vi "traffic_light.vi"() -> ()   [LabVIEW 2019]
doc: "This is a traffic light system. It realized the output with hard device or simulated device. The light has four phases."
uses:
  <vilib>/Utility/error.llb/DialogType.ctl
  <vilib>/DAQmx/write.llb/DAQmx Write (Digital 1D Bool 1Chan 1Samp).vi
  <vilib>/DAQmx/create/channels.llb/DAQmx Create Channel (DO-Digital Output).vi
  <vilib>/DAQmx/miscellaneous.llb/DAQmx Fill In Error Info.vi
panel:
  out "Delay (ms)":u32 caption="Elapsed Time (s)"
  in  "Loop Time (ms)":u32=100 max=1000 step=50
  in  "Line(s)":tag="Dev1/port0/line0:1"
  out "Phase Time (s)":dbl caption="Elapsed Time (s)" format="%.2f"
  in  "Stop Button":bool
  out "Red":bool
  out "Yellow":bool
  out "Green":bool
  # "Note & Guide\n\nLine(s)\ndevice/port/line0:2\nmyDAQ1/port0/line0:2\n\nLoop Time (ms)\n0 - 1000\nreference: 100\n\nPhase\nGreen              3s\nYellow              2s\nRed                 5s\nRed+Yellow     1s\n\nAuthor\nYufan Dong - 06.Oct.2021"
  # "Traffic Light System"
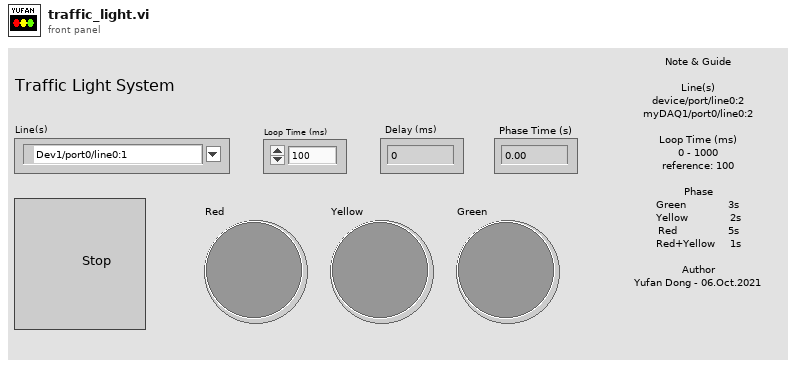
[diagram p1: front panel]
types:
  T1 = typedef "DialogType.ctl" = u16
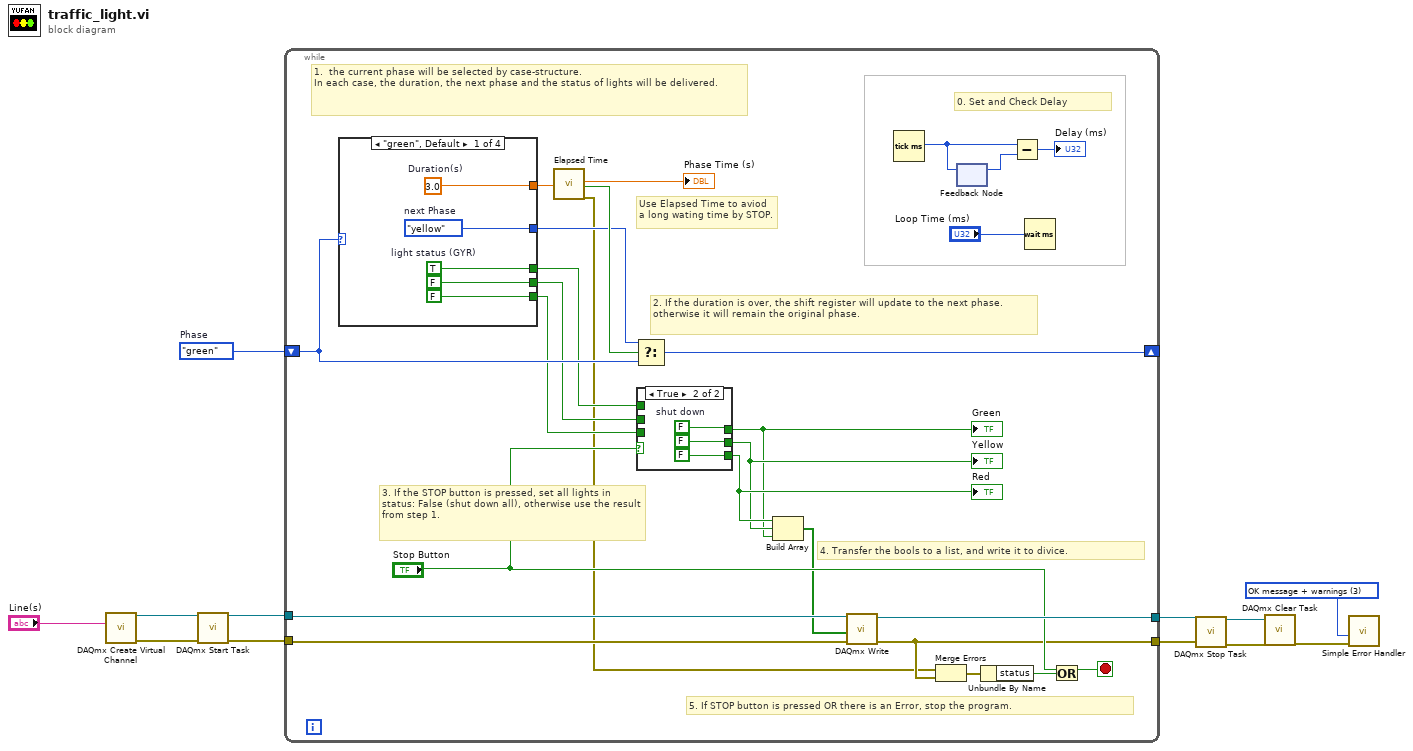
[diagram p0: block diagram]
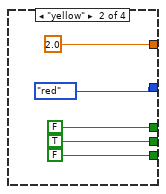
[diagram p3: hidden frame]
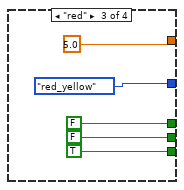
[diagram p4: hidden frame]
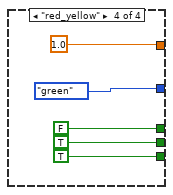
[diagram p5: hidden frame]
diagram:
  w5 = T1 3 items=["no dialog", "OK message", "continue or stop message", "OK message + warnings", "continue/stop + warnings"] ("type of dialog (OK msg:1)")
  w12 = enum16{"green", "yellow", "red", "red_yellow"}."green"  # Phase
  n1 = call-poly <vilib>:"DAQmx Create Virtual Channel.vi"("lines"="Line(s)") -> ("task out"=w8:refnum<k21>, "error out"=w9:errorcluster)  [unwired: 13 in]
  n2 = call <vilib>:"DAQmx Start Task.vi"("task/channels in"=w8, "error in"=w9) -> ("task out"=w2:refnum<k21>, "error out"=w1:errorcluster)  [unwired: 12 in]
  n3 = while {
    shift-right: [w35] -> _
    shift-left: w12 -> [w34]
    tunnel: [w28] -> w4
    tunnel: [w18] -> w3
    tunnel: w1 -> [w30]
    tunnel: w2 -> [w29]
    stop <- w27 stop-if-true
    # "Use Elapsed Time to aviod a long wating time by STOP."
    # "5. If STOP button is pressed OR there is an Error, stop the program."
    # "4. Transfer the bools to a list, and write it to divice."
    # "3. If the STOP button is pressed, set all lights in status: False (shut down all), otherwise use the result from step 1."
    # "2. If the duration is over, the shift register will update to the next phase. otherwise it will remain the original phase."
    # "1.  the current phase will be selected by case-structure. \nIn each case, the duration, the next phase and the status of lights will be delivered."
    # "0. Set and Check Delay"
    n4 = case shown="\"green\", Default" w34 {
      tunnel: [w49 2.0 5.0 1.0] -> w38
      tunnel: [FALSE TRUE FALSE TRUE] -> w25
      tunnel: [w48 FALSE FALSE FALSE] -> w26
      tunnel: [FALSE FALSE TRUE TRUE] -> w24
      tunnel: [w45 enum16{"green", "yellow", "red", "red_yellow"}."red" enum16{"green", "yellow", "red", "red_yellow"}."red_yellow" enum16{"green", "yellow", "red", "red_yellow"}."green"] -> w36
      frame "green", Default {
        w45 = enum16{"green", "yellow", "red", "red_yellow"}."yellow"  # next Phase
        w49 = 3.0  # Duration(s)
        w48 = TRUE  # light status (GYR)
      }
      frame "yellow" {
      }
      frame "red" {
      }
      frame "red_yellow" {
      }
    }
    n5 = call "Elapsed Time"("Time Target (s)"=w38) -> ("Elapsed Time (s)"=→"Phase Time (s)":dbl, "Time has Elapsed"=w37:bool, "error out"=w16:errorcluster)  [unwired: 11 in, 5 out]
    n6 = Select(t=w36, s=w37, f=w34) -> (s? t:f=w35:enum16{"green", "yellow", "red", "red_yellow"})
    n7 = case shown="True" "Stop Button" {
      tunnel: w26 -> [w41 _]
      tunnel: w25 -> [w40 _]
      tunnel: w24 -> [w39 _]
      tunnel: [w41 w42] -> w19
      tunnel: [w40 FALSE] -> w20
      tunnel: [w39 FALSE] -> w21
      frame False {
      }
      frame True {
        w42 = FALSE  # shut down
      }
    }
    "Green" <- w19
    "Yellow" <- w20
    "Red" <- w21
    n8 = Build Array(w21, w20, w19) -> (w22:bool[])
    n9 = call-poly <vilib>:"DAQmx Write.vi"("task/channels in"=w29, "data"=w22, "error in"=w30) -> ("task out"=w28:refnum<k21>, "error out"=w18:errorcluster)  [unwired: 10 in, 1 out]
    n10 = Tick Count (ms)() -> (millisecond timer value=w32:u32)
    n11 = Merge Errors(w16, w18) -> (w17:errorcluster)
    n12 = feedback-in #1(w32) -> ()
    n13 = feedback #1() -> (w33:u32)  [unwired: 1 in]
    n14 = Unbundle By Name(w17) -> ("status"=w15:bool)
    n15 = Subtract(x=w32, y=w33) -> (x-y=→"Delay (ms)":u32)
    n16 = Wait (ms)(milliseconds to wait="Loop Time (ms)") -> ()  [unwired: 1 out]
    n17 = Or(x="Stop Button", y=w15) -> (x .or. y?=w27:bool)
  }
  n18 = call <vilib>:"DAQmx Stop Task.vi"("task/channels in"=w4, "error in"=w3) -> ("task out"=w7:refnum<k21>, "error out"=w6:errorcluster)  [unwired: 12 in]
  n19 = call <vilib>:"DAQmx Clear Task.vi"("task in"=w7, "error in"=w6) -> ("error out"=w11:errorcluster)  [unwired: 13 in]
  n20 = call <vilib>:"Simple Error Handler.vi"("type of dialog (OK msg:1)"=w5, "error in (no error)"=w11) -> ()  [unwired: 3 in, 5 out]
